vi "API_Connect.vi"(8 "error in (no error)":errorcluster, 10 "Connect":bool) -> (0 "error out":errorcluster)   [LabVIEW 2015, in "Tool Module.lvlib"]
doc: "Connect or Disconnect from the tool. When the application starts, use this vi to initiate connection to the tool. If you make the Connect control False, then the tool will disconnect and then try and reconnect. So once the first connection is made, the tool always tries to connect. If you send the connect command before the tool is connected to the USB port, then the tool keeps trying to connect until a tool is attached."
uses:
  Tool Module.lvlib
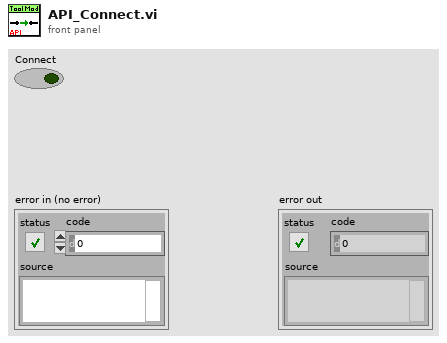
[diagram p1: front panel]
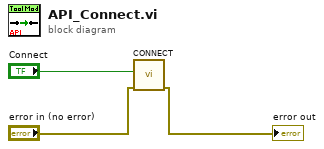
[diagram p0: block diagram]
diagram:
  n1 = call "CONNECT.vi"("error in (no error)"="error in (no error)", "Connect"="Connect") -> ("error out"=→"error out":errorcluster)  [unwired: 9 in]
